vi "resetOutput.vi"(8 "error in (no error)":errorcluster, 11 "SpinCore in":refnum<class "SpinCore.lvclass">) -> (0 "error out":errorcluster, 3 "SpinCore out":refnum<class "SpinCore.lvclass">)   [LabVIEW 2009, in "Hardware.lvlib" / "Channels.lvlib" / "SpinCore.lvclass"]
uses:
  SpinCore.lvclass
  Generic/DDSOutput.lvclass
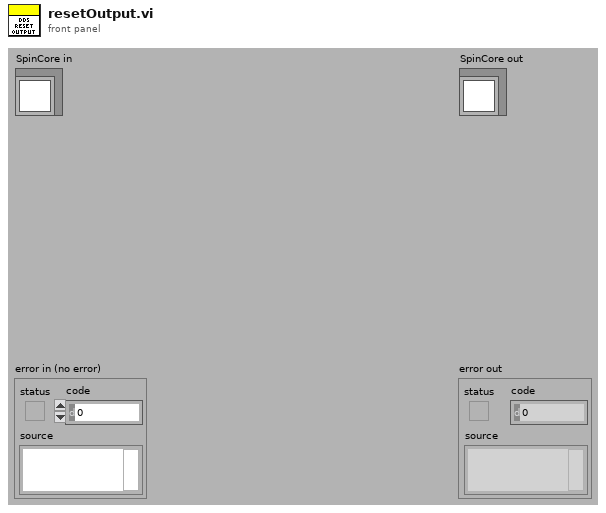
[diagram p1: front panel]
types:
  T1 = cluster{"Frequency(MHz)":dbl, "Amplitude":dbl, "Phase":dbl, "OutputForm":enum16{"Sine", "Square", "Triangle", "Arbitrary"}}[]
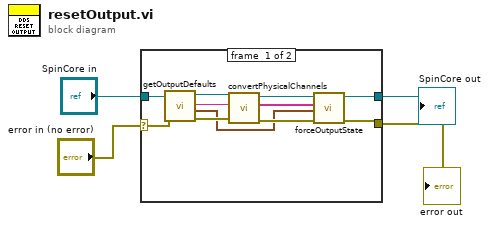
[diagram p0: block diagram]
diagram:
  n1 = case shown="No Error" "error in (no error)" {
    selector: "error in (no error)" -> [w14 w16]
    tunnel: "SpinCore in" -> [w15 w17]
    tunnel: [w13 w16] -> w2
    tunnel: [w12 w17] -> w1
    frame #0 {
      n2 = call "getOutputDefaults.vi"("error in (no error)"=w14, "DDSOutput in"=w15) -> ("error out"=w11:errorcluster, "Defaults"=w5:T1, "physical Channels"=w6:string, "DDSOutput out"=w7:refnum<class "SpinCore.lvclass">)  [unwired: 6 in]
      n3 = call "convertPhysicalChannels.vi"("error in (no error)"=w11, "physicalChannels"=w6, "DDSOutput in"=w7) -> ("error out"=w8:errorcluster, "physicalChannels"=w10:string[], "DDSOutput out"=w9:refnum<class "SpinCore.lvclass">)  [unwired: 6 in]
      n4 = call-dynamic "forceOutputState.vi"("error in (no error)"=w8, "data"=w5, "physicalChannels"=w10, "SpinCore in"=w9) -> ("error out"=w13:errorcluster, "SpinCore out"=w12:refnum<class "SpinCore.lvclass">)  [unwired: 6 in]
    }
    frame #1 {
    }
  }
  "error out" <- w2
  "SpinCore out" <- w1
